vi "sub vi - save log files V1.vi"() -> (0 "error out":errorcluster, 3 "network dir":string)   [LabVIEW 2017]
uses:
  program files/Global 1.vi
panel:
  out "file dir":string
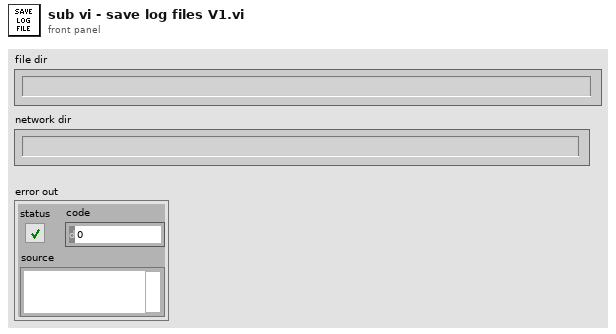
[diagram p1: front panel]
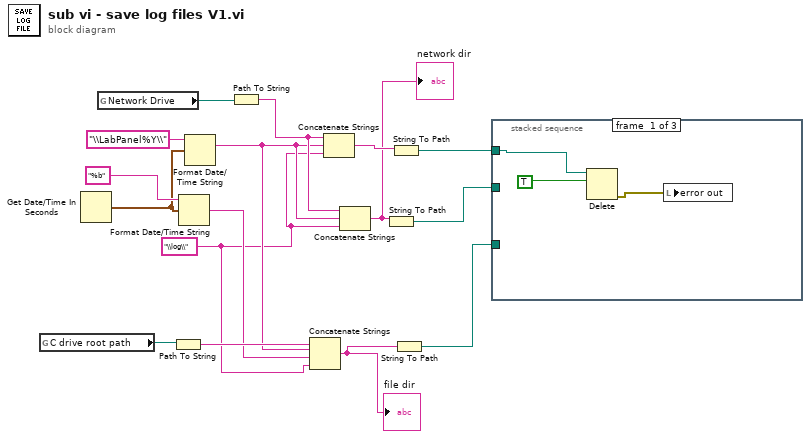
[diagram p0: block diagram]
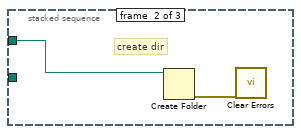
[diagram p2: hidden frame]
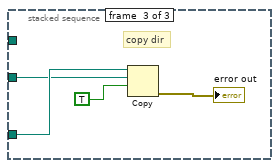
[diagram p3: hidden frame]
diagram:
  w2 = "\\log\\"
  n1 = global read "Global 1.vi" "C drive root path"() -> (w11:path)
  n2 = Get Date/Time In Seconds() -> (seconds since 1Jan1904=w13:timestamp)
  n3 = global read "Global 1.vi" "Network Drive"() -> (w14:path)
  n4 = Path To String(path=w11) -> (string=w12:string)
  n5 = Format Date/Time String(time format string (%c)="%b", seconds (now)=w13) -> (date/time string=w3:string)  [unwired: 1 in]
  n6 = Format Date/Time String(time format string (%c)="\\LabPanel%Y\\", seconds (now)=w13) -> (date/time string=w5:string)  [unwired: 1 in]
  n7 = Path To String(path=w14) -> (string=w6:string)
  n8 = Concatenate Strings(w12, w5, w3, w2) -> (w9:string)
  "file dir" <- w9
  n9 = Concatenate Strings(w6, w5, w2) -> (w10:string)
  n10 = Concatenate Strings(w6, w5, w2) -> (w1:string)
  "network dir" <- w1
  n11 = String To Path(string=w1) -> (path=w4:path)
  n12 = String To Path(string=w10) -> (path=w8:path)
  n13 = String To Path(string=w9) -> (path=w7:path)
  n14 = stacked-sequence {
    tunnel: w8 -> [w19 w20 _]
    tunnel: w7 -> [_ _ w24]
    tunnel: w4 -> [_ _ w22]
    frame #0 {
      n15 = Delete(path (use dialog)=w19, entire hierarchy (F)=TRUE) -> (error out=w18:errorcluster)  [unwired: 3 in, 2 out]
      n16 = local write "error out"(w18) -> ()
    }
    frame #1 {
      # "create dir"
      n17 = Create Folder(path (use dialog)=w20) -> (error out=w21:errorcluster)  [unwired: 2 in, 2 out]
      n18 = call <vilib>:"Clear Errors.vi"("error in (no error)"=w21) -> ()  [unwired: 5 in, 2 out]
    }
    frame #2 {
      # "copy dir"
      n19 = Copy(9:TRUE, 10:w22, 11:w24) -> (0:→"error out":errorcluster)  [unwired: 2 in, 2 out]
    }
  }
